vi "Collapse Channels Array into Blocks.vi"(11 "channel configurations in":T1[](array[typedef]) {"count" format="%d bytes"}) -> (3 "channel configurations out":T1[](array[typedef]) {"count" format="%d bytes"})   [LabVIEW 2017, in "Data Sharing Framework Core.lvlib" / "Data Sharing Framework Engine.lvlib" / "Framework Configuration.lvclass"]
uses:
  Framework Configuration.lvclass
  Configuration/1.0.0/Public/Controls/DSF Engine Channel Configuration.ctl
  Configuration/1.0.0/Public/Controls/DSF Data Type.ctl
  Configuration/1.0.0/Public/Controls/DSF Settings Info.ctl
  Datatype Size Methods/Get Datatype Size.vi
  Data Sharing Framework Engine.lvlib
  Configuration/1.0.0/Data Sharing Framework Configuration.lvlib
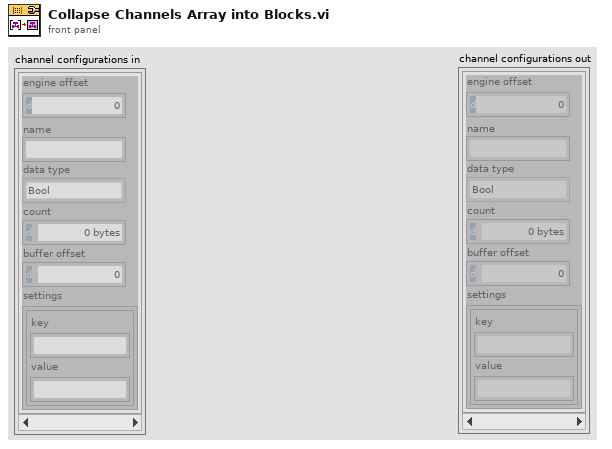
[diagram p1: front panel]
types:
  T1 = typedef "Data Sharing Framework Core.lvlib/Data Sharing Framework Configuration.lvlib/DSF Engine Channel Configuration.ctl" = cluster{"engine offset":u64, "name":string, "data type":T2, "count":u64, "buffer offset":u64, "settings":T3}
  T2 = typedef "Data Sharing Framework Core.lvlib/Data Sharing Framework Configuration.lvlib/DSF Data Type.ctl" = enum8{"Bool", "SGL", "DBL", "I8", "I16", "I32", "I64", "U8", "U16", "U32", "U64"}
  T3 = typedef "Data Sharing Framework Core.lvlib/Data Sharing Framework Configuration.lvlib/DSF Settings Info.ctl" = cluster{"key":string, "value":string}[]
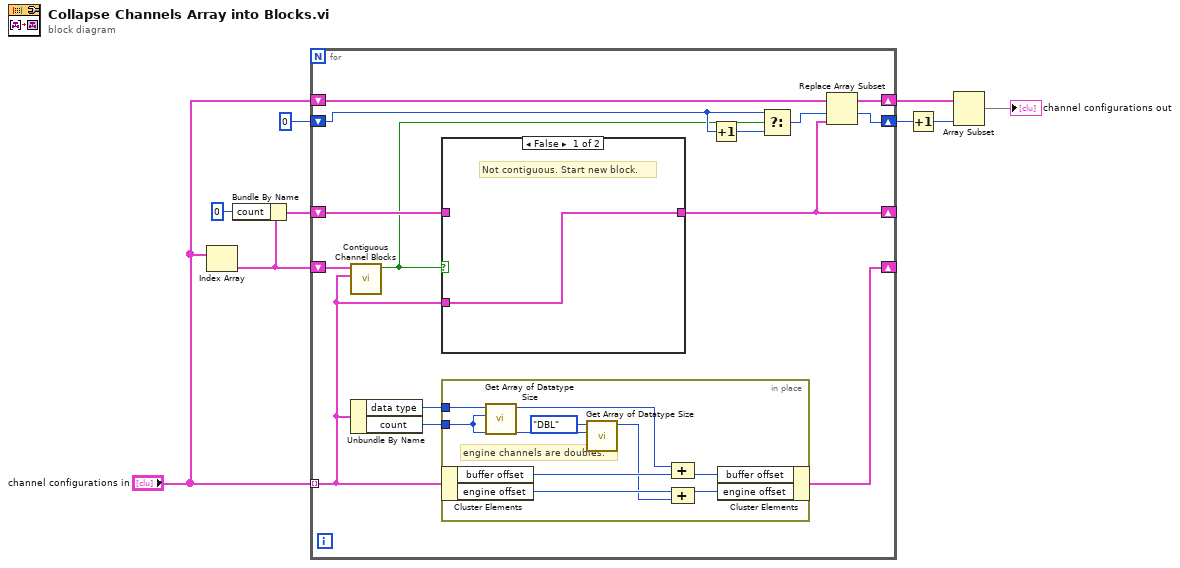
[diagram p0: block diagram]
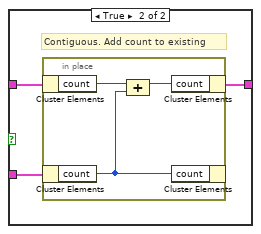
[diagram p2: hidden frame]
diagram:
  n1 = Index Array(array="channel configurations in") -> (element=w4:T1)  [unwired: 1 in]
  n2 = Bundle By Name(cluster=w4, "count"=u64 0) -> (w5:T1)
  n3 = for {
    tunnel: "channel configurations in" -> [w17] mode=indexing
    shift-right: [w22] -> w8
    shift-left: "channel configurations in" -> [w10]
    shift-right: [w21] -> _
    shift-left: w4 -> [w18]
    shift-right: [w13] -> w2
    shift-left: 0 -> [w14]
    shift-right: [w11] -> _
    shift-left: w5 -> [w16]
    n4 = call "Contiguous Channel Blocks.vi"("current channel block"=w17, "expected channel block"=w18) -> ("contiguous?"=w12:bool)  [unwired: 9 in]
    n5 = Unbundle By Name(w17) -> ("data type"=w20:T2, "count"=w19:u64)
    n6 = case shown="False" w12 {
      tunnel: w17 -> [w32 w35]
      tunnel: w16 -> [_ w34]
      tunnel: [w32 w33] -> w11
      frame False {
        # "Not contiguous. Start new block."
      }
      frame True {
        # "Contiguous. Add count to existing"
        n7 = in-place {
          n8 = in-place-cluster #1(w34) -> ("count"=w38:u64)
          n9 = in-place-cluster #2(w35) -> ("count"=w36:u64)
          n10 = Compound Arithmetic op=ADD(w38, w36) -> (w37:u64)
          n11 = in-place-cluster #1("count"=w37) -> (w33:T1)
          n12 = in-place-cluster #2("count"=w36) -> ()  [unwired: 1 out]
        }
      }
    }
    n13 = in-place {
      in-place-border: w20 -> [w24]
      in-place-border: w19 -> [w25]
      # "engine channels are doubles."
      n14 = in-place-cluster #3(w17) -> ("buffer offset"=w31:u64, "engine offset"=w29:u64)
      n15 = call "Get Array of Datatype Size.vi"("count"=w25, "data type"=w24) -> ("size in bytes"=w26:u64)  [unwired: 9 in]
      n16 = call "Get Array of Datatype Size.vi"("count"=w25, "data type"=DSF_Data_Type."DBL") -> ("size in bytes"=w23:u64)  [unwired: 9 in]
      n17 = Compound Arithmetic op=ADD(w26, w31) -> (w30:u64)
      n18 = Compound Arithmetic op=ADD(w29, w23) -> (w28:u64)
      n19 = in-place-cluster #3("buffer offset"=w30, "engine offset"=w28) -> (w21:T1)
    }
    n20 = Increment(x=w14) -> (x+1=w15:i32)
    n21 = Select(t=w14, s=w12, f=w15) -> (s? t:f=w13:i32)
    n22 = Replace Array Subset(array=w10, new element=w11, index=w13) -> (w22:T1[])
  }
  n23 = Increment(x=w2) -> (x+1=w1:i32)
  n24 = Array Subset(array=w8, length=w1) -> (→"channel configurations out":T1[])  [unwired: 1 in]
